vi "Show GPIB Config Panel.vi"(1 "error in (no error)":errorcluster, 2 "Array":refnum<vi>[](array[refnum])) -> (0 "error out":errorcluster)   [LabVIEW 2021]
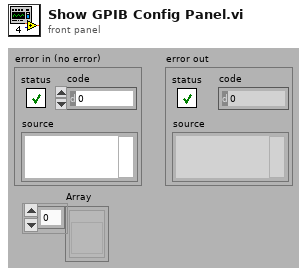
[diagram p1: front panel]
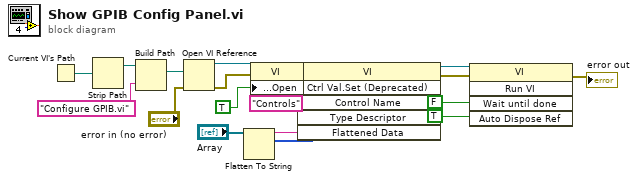
[diagram p0: block diagram]
diagram:
  n1 = Current VI's Path() -> (path=w16:path)
  n2 = Strip Path(path=w16) -> (stripped path=w13:path)  [unwired: 1 out]
  n3 = Build Path(base path=w13, name or relative path="Configure GPIB.vi") -> (appended path=w15:path)
  n4 = Open VI Reference(vi path=w15, error in (no error)="error in (no error)") -> (vi reference=w19:refnum<vi>, error out=w17:errorcluster)  [unwired: 4 in]
  n5 = Flatten To String(anything="Array") -> (data string=w2:string, type string=w3:i16[])  [unwired: 3 in, 1 out]
  n6 = property class="VI"(reference=w19, error in=w17, "Front Panel Window:Open"=TRUE) -> (reference out=w6:refnum<vi>, error out=w12:errorcluster)
  n7 = invoke class="VI" method="Ctrl Val.Set (Deprecated)"(reference=w6, error in=w12, "Control Name"="Controls", "Type Descriptor"=w3, "Flattened Data"=w2) -> (reference out=w5:refnum<vi>, error out=w7:errorcluster)  [unwired: 1 in, 4 out]
  n8 = invoke class="VI" method="Run VI"(reference=w5, error in=w7, "Wait until done"=FALSE, "Auto Dispose Ref"=TRUE) -> (error out=→"error out":errorcluster)  [unwired: 1 in, 4 out]
